vi "OP_SubVI.vi"(0 "High Byte":u8, 3 "Low Byte":u8) -> (7 "Oil Pressure":u16)   [LabVIEW 2012]
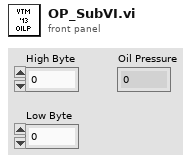
[diagram p1: front panel]
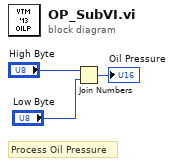
[diagram p0: block diagram]
diagram:
  # "Process Oil Pressure"
  n1 = Join Numbers(hi="High Byte", lo="Low Byte") -> ((hi.lo)=→"Oil Pressure":u16)
